vi "getXAxisConversionType.vi"(6 "Delay between send and receive [ms]":i32=100, 8 "error in (no error)":errorcluster, 11 "CCD in":refnum<class "CCD.lvclass">) -> (0 "error out":errorcluster, 2 "x axis conversion type":T1, 3 "CCD out":refnum<class "CCD.lvclass">)   [LabVIEW 2023, in "CCD.lvclass"]
uses:
  CCD.lvclass
  CCD.lvclass/CCD.ctl
  20f7d3bd-08ac-4524-9bed-df36c1da25a0.vi
  a21955fc-e3a0-4e36-8495-41f1bfac7860.vi
  GenericDevice/GenericDevice.lvclass
  XAxisConversionType.ctl
  <vilib>/IlluminatedG/lv-web-crypto/lv-json/JSON/JSON.lvlib
  XAxisConversionTypeEnum.ctl
panel:
  # "Connector Pane"
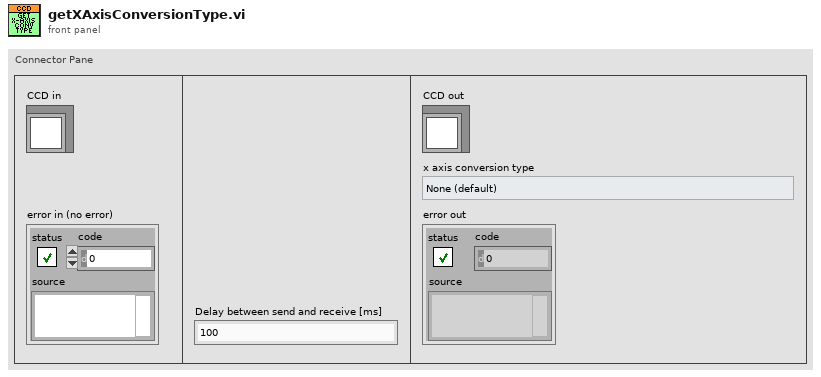
[diagram p1: front panel]
types:
  T1 = typedef "CCD.lvclass/XAxisConversionTypeEnum.ctl" = enum16{"None (default)", "CCD FIT parameters contained in the CCD firmware", "Mono Wavelength parameters contained in the icl_settings.ini file"}
  T2 = typedef "CCD.lvclass/XAxisConversionType.ctl" = cluster{"type":u16}
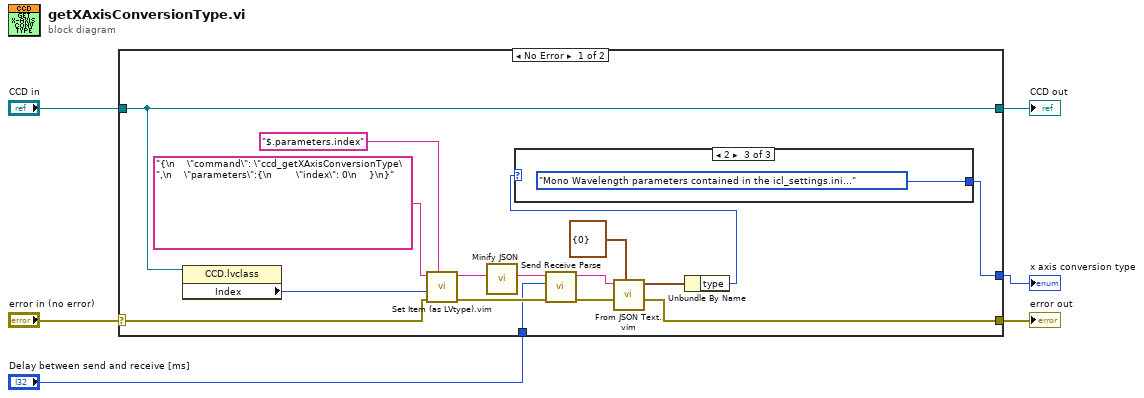
[diagram p0: block diagram]
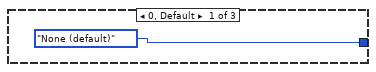
[diagram p2: hidden frame]
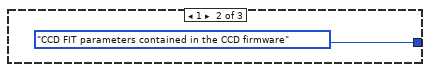
[diagram p3: hidden frame]
diagram:
  n1 = case shown="No Error" "error in (no error)" {
    selector: "error in (no error)" -> [w18 w27]
    tunnel: [w17 w27] -> w5
    tunnel: [w20 w26] -> w3
    tunnel: "CCD in" -> [w20 w26]
    tunnel: [w9 _] -> w2
    tunnel: "Delay between send and receive [ms]" -> [w7 _]
    frame No Error {
      n2 = property class="CCD.lvclass"(reference=w20) -> ("Index"=w19:i32)  [unwired: 1 in, 2 out]
      n3 = call "Set Item (as LVtype).vim"("$Path or Item Name"="$.parameters.index", "error in (no error)"=w18, "Anything"=w19, "JSON"="{\n    \"command\": \"ccd_getXAxisConversionType\",\n    \"parameters\":{\n        \"index\": 0\n    }\n}") -> ("error out"=w15:errorcluster, "<JSON>"=w11:string)  [unwired: 4 in, 1 out]
      n4 = call <vilib>:"Minify JSON.vi"("JSON String"=w11) -> ("Minified JSON"=w10:string)  [unwired: 10 in]
      n5 = call "Send Receive Parse.vi"("error in"=w15, "Delay between send and receive [ms]"=w7, "<JSON>"=w10) -> ("error out"=w14:errorcluster, "results-JSON string"=w16:string)  [unwired: 6 in, 1 out]
      n6 = call "From JSON Text.vim"("Data Type and Default Value"=T2 {"type"=0} ("XAxisConversionType"), "error in (no error)"=w14, "JSON"=w16) -> ("error out"=w17:errorcluster, "Data out"=w12:T2)  [unwired: 7 in]
      n7 = Unbundle By Name(w12) -> ("type"=w8:u16)
      n8 = case shown="2" w8 {
        tunnel: [XAxisConversionTypeEnum."None (default)" ("type") XAxisConversionTypeEnum."CCD FIT parameters contained in the CCD firmware" ("type") XAxisConversionTypeEnum."Mono Wavelength parameters contained in the icl_settings.ini file" ("type")] -> w9
        frame 0, Default {
        }
        frame 1 {
        }
        frame 2 {
        }
      }
    }
    frame Error {
    }
  }
  "error out" <- w5
  "CCD out" <- w3
  "x axis conversion type" <- w2
